vi "CleanSurface_3d.vi"(7 "Rep. Rate (Hz)":dbl=1000.0 min=0.0 max=34.0, 10 "Start Position":dbl[](array[numeric]) min=0.0 max=34.0) -> (0 "BNC_Ctrl":bool, 1 "start/end points":cluster{dbl, dbl, dbl}[][](array[cluster]), 2 "Canceled":bool, 5 "ImageParameter":T1)   [LabVIEW 2013]
uses:
  ImagingMS/ImageConvPara_3d.ctl
panel:
  in  "Z Steps":i32=1 min=0 max=34
  out "EstimatedTime":dbl caption="Estimated Time (min)" min=0.0 max=34.0
  in  "Speed":dbl=10.0 min=0.0 max=34.0
  in  "Apply":bool
  in  "Cancel":bool
  in  "Run":bool
  out "XY Graph":cluster{dbl, dbl, "X StepWidth":dbl}[](graph)
  out "Y Size (mm)":dbl min=0.0 max=34.0
  out "X Size (mm)":dbl min=0.0 max=34.0
  in  "Y Steps":i32=120 min=0 max=34
  in  "X Size":dbl=1.2 min=0.0 max=34.0
  in  "Y StepWidth":dbl=0.01 min=0.0 max=34.0
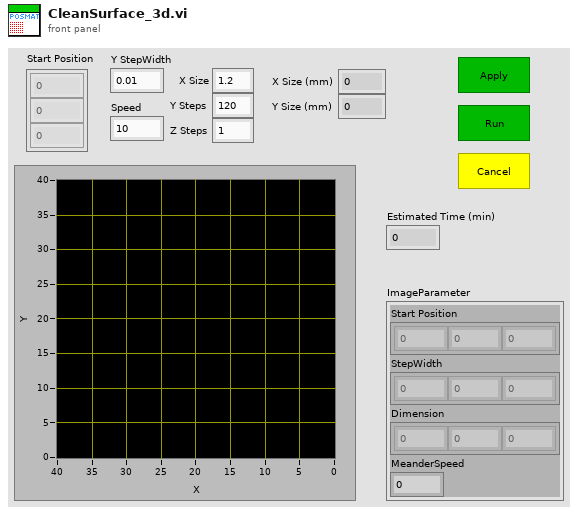
[diagram p1: front panel]
types:
  T1 = typedef "ImageConvPara_3d.ctl" = cluster{"Start Position":dbl[], "StepWidth":dbl[], "Dimension":i32[], "MeanderSpeed":dbl}
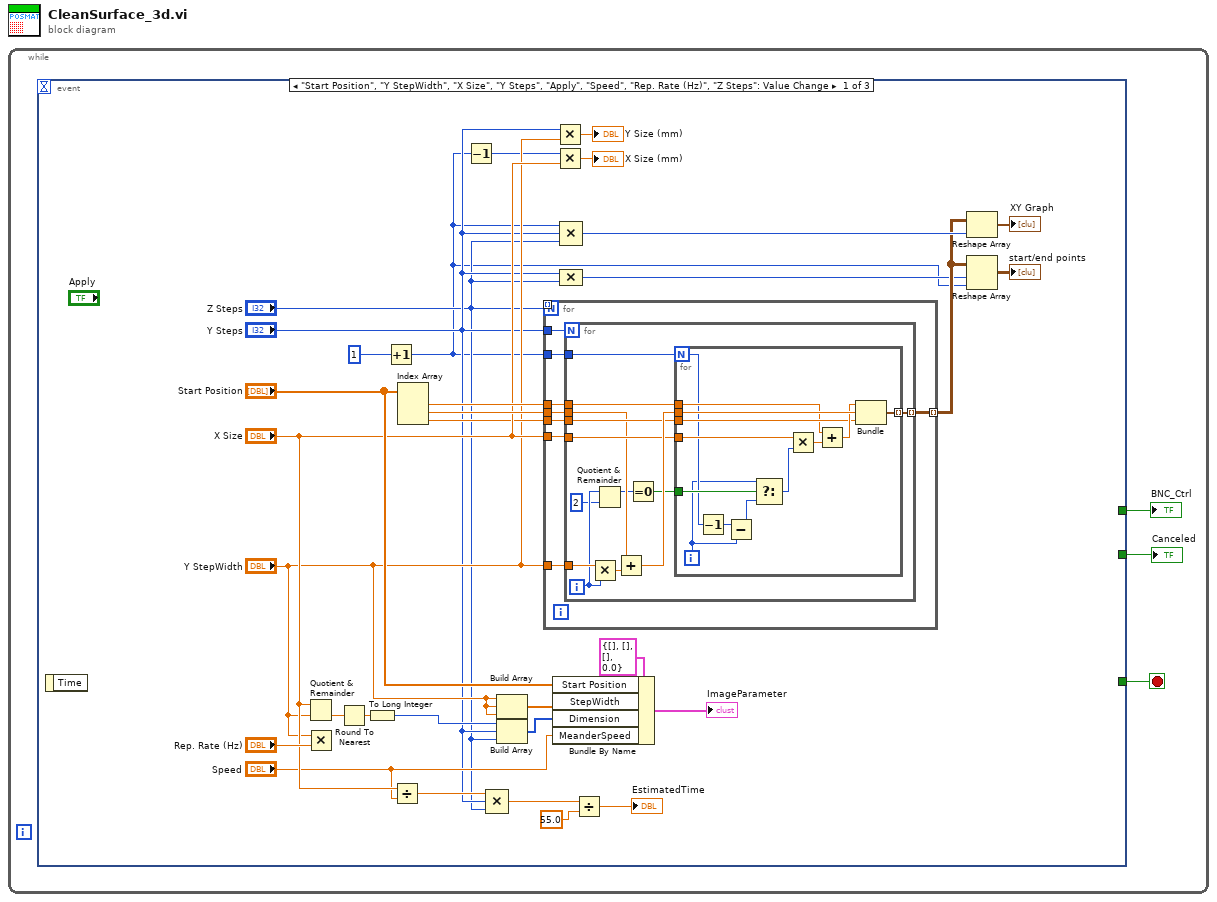
[diagram p0: block diagram]
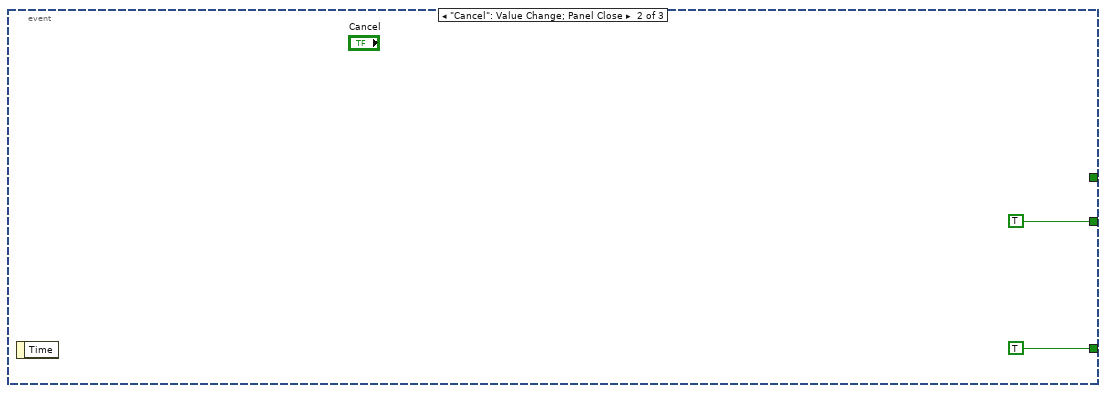
[diagram p2: hidden frame]
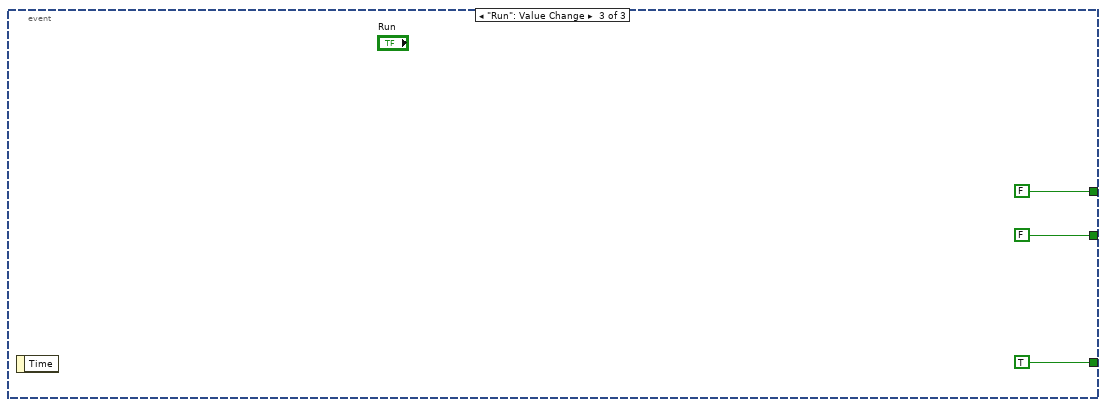
[diagram p3: hidden frame]
diagram:
  n1 = while {
    stop <- w3 stop-if-true
    n2 = event shown="[0] \"Start Position\", \"Y StepWidth\", \"X Size\", \"Y Steps\", \"Apply\", \"Speed\", \"Rep. Rate (Hz)\", \"Z Steps\": Value Change" {
      selector: _ -> [_ _ _]
      dyn-events: _ -> [_ _ _]
      timeout: _ -> [_ _ _]
      tunnel: [_ TRUE TRUE] -> w3
      tunnel: [_ TRUE ("Canceled") FALSE ("Canceled")] -> w2
      tunnel: [_ _ FALSE ("Imaging?")] -> w1
      event "Start Position", "Y StepWidth", "X Size", "Y Steps", "Apply", "Speed", "Rep. Rate (Hz)", "Z Steps": Value Change {
        n3 = event-data() -> ()  [unwired: 1 in, 1 out]
        n4 = Quotient & Remainder(x="X Size", y="Y StepWidth") -> (floor(x/y)=w24:dbl)  [unwired: 1 out]
        n5 = Multiply(x="Y StepWidth", y="Rep. Rate (Hz)") -> ()  [unwired: 1 out]
        n6 = Round To Nearest(number=w24) -> (nearest integer value=w16:dbl)
        n7 = To Long Integer(number=w16) -> (32bit integer=w17:i32)
        n8 = Increment(x=1) -> (x+1=w4:i32)
        n9 = Divide(x="X Size", y="Speed") -> (x/y=w11:dbl)
        n10 = Index Array(array="Start Position") -> (element #1=w34:dbl, element #2=w33:dbl, element #3=w18:dbl)  [unwired: 3 in]
        n11 = Decrement(x=w4) -> (x-1=w8:i32)
        n12 = Compound Arithmetic op=MULTIPLY(w11, "Y Steps", "Z Steps") -> (w21:dbl)
        n13 = Build Array("Y StepWidth", "Y StepWidth", "Y StepWidth") -> (w27:dbl[])
        n14 = Build Array(w17, "Y Steps", "Z Steps") -> (w26:i32[])
        n15 = for {
          N: "Z Steps" -> [w36]
          tunnel: w34 -> [w43]
          tunnel: w33 -> [w42]
          tunnel: w4 -> [w41]
          tunnel: [w35] -> w10 mode=indexing
          tunnel: "Y StepWidth" -> [w40]
          tunnel: "X Size" -> [w39]
          tunnel: w18 -> [w38]
          tunnel: "Y Steps" -> [w37]
          tunnel: [w36] -> _ mode=indexing
          n16 = for {
            N: w37 -> [_]
            tunnel: w42 -> [w48]
            tunnel: w40 -> [w49]
            tunnel: w39 -> [w52]
            tunnel: w41 -> [w54]
            tunnel: [w53] -> w35 mode=indexing
            tunnel: w38 -> [w50]
            tunnel: w43 -> [w51]
            i -> [w46]
            n17 = Multiply(x=w49, y=w46) -> (x*y=w56:dbl)
            n18 = Quotient & Remainder(x=w46, y=2) -> (x-y*floor(x/y)=w47:i32)  [unwired: 1 out]
            n19 = Add(x=w48, y=w56) -> (x+y=w55:dbl)
            n20 = Equal To 0?(x=w47) -> (x = 0?=w44:bool)
            n21 = for {
              N: w54 -> [w60]
              tunnel: w52 -> [w68]
              tunnel: w51 -> [w63]
              tunnel: w55 -> [w66]
              tunnel: [w67] -> w53 mode=indexing
              tunnel: w50 -> [w64]
              tunnel: w44 -> [w62]
              i -> [w59]
              n22 = Decrement(x=w60) -> (x-1=w61:i32)
              n23 = Subtract(x=w61, y=w59) -> (x-y=w58:i32)
              n24 = Select(t=w59, s=w62, f=w58) -> (s? t:f=w57:i32)
              n25 = Multiply(x=w68, y=w57) -> (x*y=w69:dbl)
              n26 = Add(x=w63, y=w69) -> (x+y=w65:dbl)
              n27 = Bundle(w65, w66, "X StepWidth"=w64) -> (w67:cluster{dbl, dbl, "X StepWidth":dbl})  [unwired: 1 in]
            }
          }
        }
        n28 = Bundle By Name(cluster=T1 {"Start Position"=[], "StepWidth"=[], "Dimension"=[], "MeanderSpeed"=0.0} ("ImageParameter 2"), "Start Position"="Start Position", "StepWidth"=w27, "Dimension"=w26, "MeanderSpeed"="Speed") -> (→"ImageParameter":T1)
        n29 = Multiply(x="Y Steps", y="Y StepWidth") -> (x*y=→"Y Size (mm)":dbl)
        n30 = Multiply(x=w8, y="X Size") -> (x*y=→"X Size (mm)":dbl)
        n31 = Compound Arithmetic op=MULTIPLY(w4, "Y Steps", "Z Steps") -> (w30:i32)
        n32 = Compound Arithmetic op=MULTIPLY("Y Steps", "Z Steps") -> (w5:i32)
        n33 = Divide(x=w21, y=55.0) -> (x/y=→"EstimatedTime":dbl)
        n34 = Reshape Array(w10, w30) -> (→"XY Graph":cluster{dbl, dbl, "X StepWidth":dbl}[])
        n35 = Reshape Array(w10, w5, w4) -> (→"start/end points":cluster{dbl, dbl, "X StepWidth":dbl}[][])
      }
      event "Cancel": Value Change; Panel Close {
        n36 = event-data() -> ()  [unwired: 1 in, 1 out]
      }
      event "Run": Value Change {
        n37 = event-data() -> ()  [unwired: 1 in, 1 out]
      }
    }
    "Canceled" <- w2
    "BNC_Ctrl" <- w1
  }
